vi "hw2-3 topVI.vi"() -> ()   [LabVIEW 2014]
panel:
  out "top 10 scores":dbl[](array[numeric])
  out "XY Graph":cluster{i32[], "top 10 scores":dbl[]}(graph)
  out "Table":string[][](table)
  out "generated sores":cluster{"score generator":dbl, i32}[](array[cluster])
  in  "Maximum Score":dbl=80.0
  in  "Minmium Score":dbl=20.0
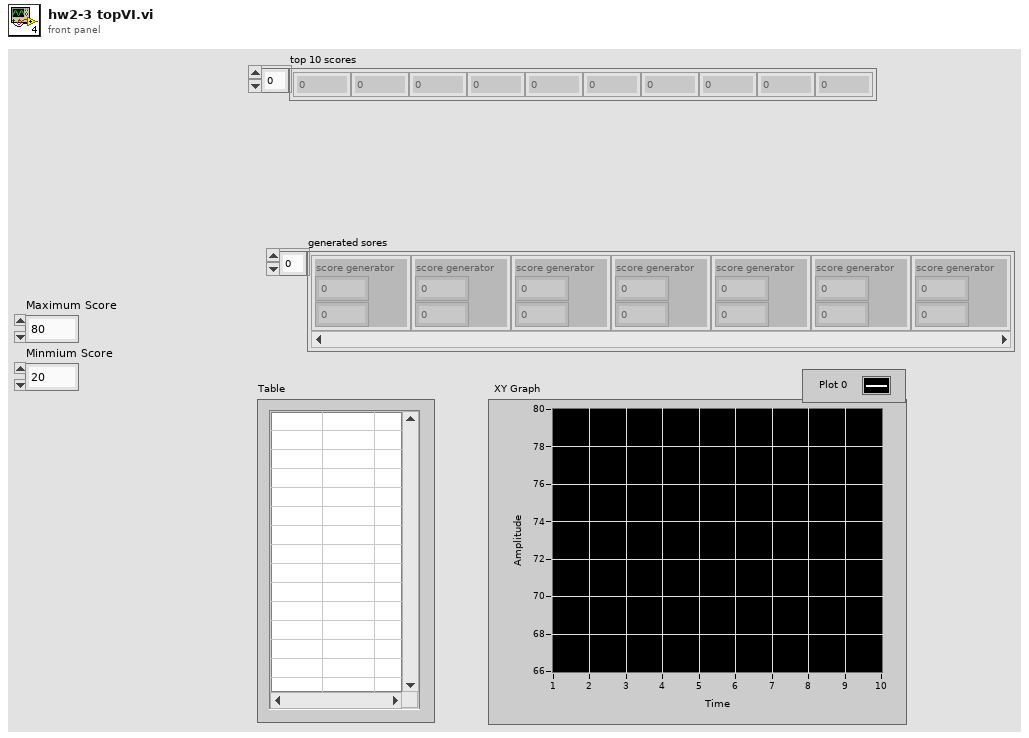
[diagram p1: front panel]
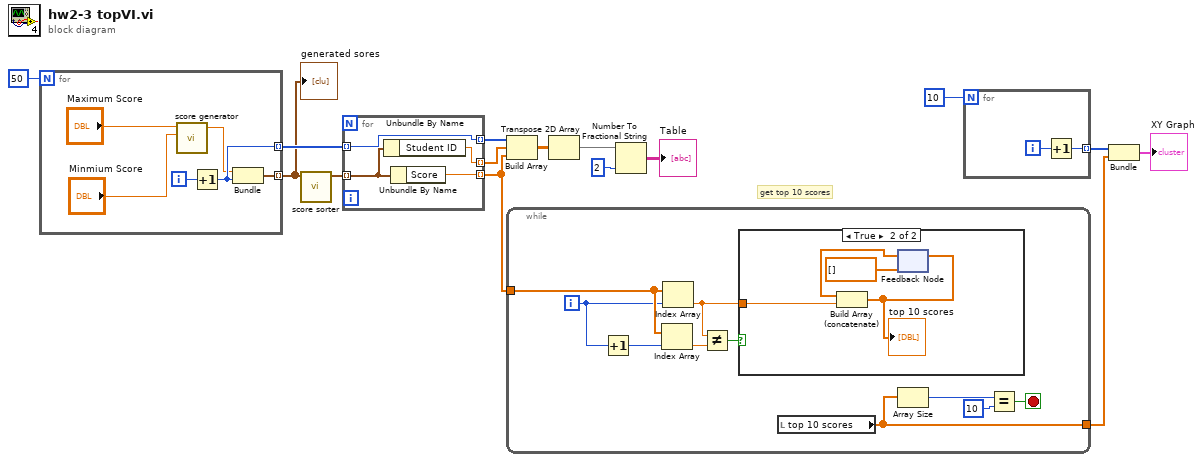
[diagram p0: block diagram]
diagram:
  # "get top 10 scores"
  n1 = for {
    N: 50 ("Number of Students") -> [_]
    tunnel: [w20] -> w3 mode=indexing
    tunnel: [w19] -> w14 mode=indexing
    i -> [w21]
    n2 = call "score generator.vi"("min score"="Minmium Score", "max score"="Maximum Score") -> ("generated score"=w18:dbl)  [unwired: 4 in]
    n3 = Increment(x=w21) -> (x+1=w19:i32)
    n4 = Bundle("generated score"=w18, w19) -> (w20:cluster{"generated score":dbl, i32})  [unwired: 1 in]
  }
  "generated sores" <- w3
  n5 = call "score sorter.vi"("array of cluster"=w3) -> ("sorted by score"=w4:cluster{"Score":dbl, "Student ID":dbl}[])  [unwired: 10 in]
  n6 = for {
    tunnel: w4 -> [w25] mode=indexing
    tunnel: [w24] -> w1 mode=indexing
    tunnel: [w23] -> w12 mode=indexing
    tunnel: w14 -> [w22] mode=indexing
    tunnel: [w22] -> w13 mode=indexing
    n7 = Unbundle By Name(w25) -> ("Student ID"=w23:dbl)
    n8 = Unbundle By Name(w25) -> ("Score"=w24:dbl)
  }
  n9 = Build Array(w13, w12, w1) -> (w11:dbl[][])
  n10 = while {
    tunnel: w1 -> [w35]
    tunnel: [w26] -> w2
    i -> [w34]
    stop <- w27 stop-if-true
    n11 = Increment(x=w34) -> (x+1=w33:i32)
    n12 = Index Array(array=w35, index=w33) -> (element=w32:dbl)
    n13 = Index Array(array=w35, index=w34) -> (element=w30:dbl)
    n14 = Not Equal?(x=w30, y=w32) -> (x != y?=w31:bool)
    n15 = case shown="True" w31 {
      tunnel: w30 -> [_ w39]
      frame False {
      }
      frame True {
        n16 = feedback #1(dbl[] []) -> (w38:dbl[])
        n17 = Build Array (concatenate)(w38, w39) -> (w36:dbl[])
        "top 10 scores" <- w36
        n18 = feedback-in #1(w36) -> ()
      }
    }
    n19 = local read "top 10 scores"() -> (w26:dbl[])
    n20 = Array Size(array=w26) -> (size(s)=w29:i32)
    n21 = Equal?(x=w29, y=10) -> (x = y?=w27:bool)
  }
  n22 = Transpose 2D Array(2D array=w11) -> (transposed array=w10:dbl[][])
  n23 = Number To Fractional String(number=w10, precision (6)=2) -> (F-format string=→"Table":string[][])  [unwired: 2 in]
  n24 = for {
    N: 10 -> [_]
    tunnel: [w40] -> w5 mode=indexing
    i -> [w41]
    n25 = Increment(x=w41) -> (x+1=w40:i32)
  }
  n26 = Bundle(w5, "top 10 scores"=w2) -> (→"XY Graph":cluster{i32[], "top 10 scores":dbl[]})  [unwired: 1 in]
